vi "write system hardware reference.vi"(8 "error in":errorcluster, 10 "system hardware ref":refnum<data-value>, 11 "Controller in":refnum<class "Controller.lvclass">) -> (0 "error out":errorcluster, 3 "Controller out":refnum<class "Controller.lvclass">)   [LabVIEW 2016, in "SMI.lvlib" / "Controller.lvclass"]
uses:
  Controller.lvclass
  Controller.lvclass/Controller.ctl
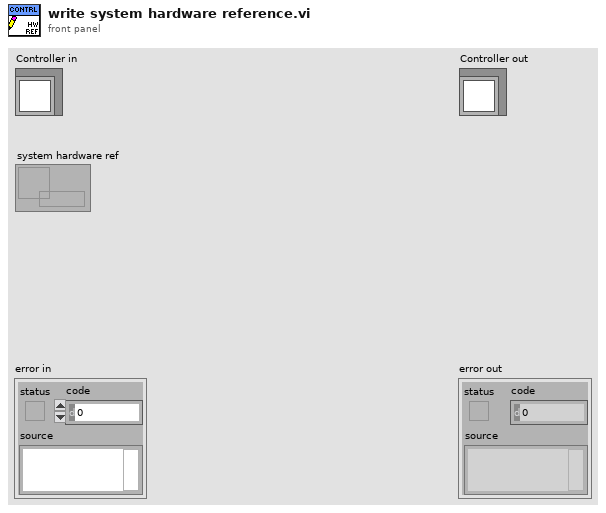
[diagram p1: front panel]
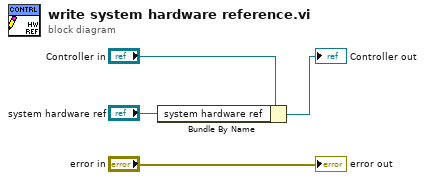
[diagram p0: block diagram]
diagram:
  n1 = Bundle By Name(cluster="Controller in", "system hardware ref"="system hardware ref") -> (→"Controller out":refnum<class "Controller.lvclass">)
  "error out" <- "error in"
